vi "Test.vi"   [LabVIEW 2025, in "Lib2.lvlib" / "Class.lvclass"]
uses:
  Class.lvclass
  Class.lvclass/Class.ctl
  Lib1/Class/Class.lvclass
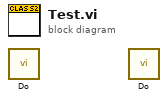
[diagram p0: block diagram]
diagram:
  n1 = call "Do.vi"() -> ()  [unwired: 12 in]
  n2 = call "Do.vi"() -> ()  [unwired: 12 in]
